vi "OpenViServer.vi"(8 "error in (no error)":errorcluster, 11 "vi path":path) -> (0 "error out":errorcluster, 3 "VI Refnum":refnum<vi>)   [LabVIEW 2015]
panel:
  in  "Activate?":bool=TRUE
  in  "State":T1(ring)=enum."Standard"
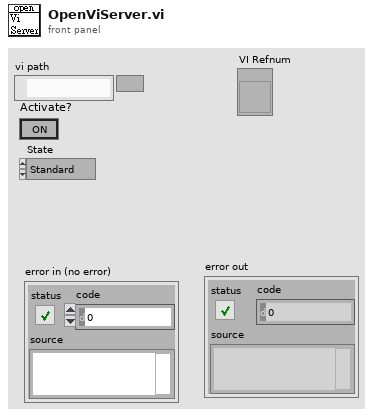
[diagram p1: front panel]
types:
  T1 = enum32{"Invalid", "Standard", "Closed", "Hidden", "Minimized", "Maximized"}
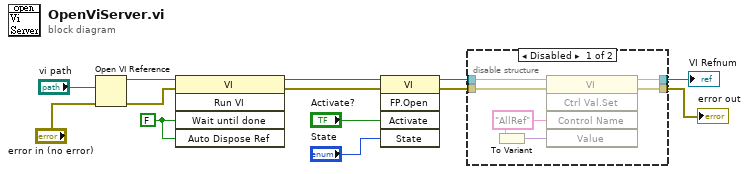
[diagram p0: block diagram]
diagram:
  w11 = FALSE ("Wait until done")
  n1 = Open VI Reference(vi path="vi path", error in (no error)="error in (no error)") -> (vi reference=w6:refnum<vi>, error out=w12:errorcluster)  [unwired: 4 in]
  n2 = invoke class="VI" method="Run VI"(reference=w6, error in=w12, "Wait until done"=w11, "Auto Dispose Ref"=w11) -> (reference out=w9:refnum<vi>, error out=w10:errorcluster)  [unwired: 1 in, 3 out]
  n3 = invoke class="VI" method="FP.Open"(reference=w9, error in=w10, "Activate"="Activate?", "State"="State") -> (reference out=w13:refnum<vi>, error out=w7:errorcluster)  [unwired: 1 in, 3 out]
  n4 = disable-structure shown="Disabled" {
    disable-tunnel: w13 -> [w19 w21]
    disable-tunnel: w7 -> [w18 w20]
    disable-tunnel: [w16 w21] -> w3
    disable-tunnel: [w15 w20] -> w1
    frame Disabled {
      w14 = "AllRef" ("Control Name")
      n5 = To Variant(anything=w14) -> (Variant=w17:variant)
      n6 = invoke class="VI" method="Ctrl Val.Set"(reference=w19, error in=w18, "Control Name"=w14, "Value"=w17) -> (reference out=w16:refnum<vi>, error out=w15:errorcluster)  [unwired: 1 in, 3 out]
    }
    frame Enabled {
    }
  }
  "VI Refnum" <- w3
  "error out" <- w1
